vi "chooseKeeperPlay.vi"(8 "error in (no error)":errorcluster, 11 "Game in":refnum<class "Game.lvclass">) -> (0 "error out":errorcluster, 3 "Game out":refnum<class "Game.lvclass">)   [LabVIEW 2023, in "Game.lvclass"]
uses:
  Game.lvclass
  Game.lvclass/Game.ctl
  Team_class/Team.lvclass/Team.ctl
  HaltPlay_class/HaltPlay.lvclass
  ZigZagPlay_class/ZigZagPlay.lvclass
  TestPlay_class/TestPlay.lvclass
  TimeoutPlay_class/TimeoutPlay.lvclass
  Team_class/KeeperPlay.ctl
  Read KeeperTeam.vi
  Team_class/Read KeeperPlay.vi
  Read AllyRef.vi
  Team_class/Write KeeperPlay.vi
  Write AllyRef.vi
  Write KeeperTeam.vi
  Ally_class/Ally.lvclass
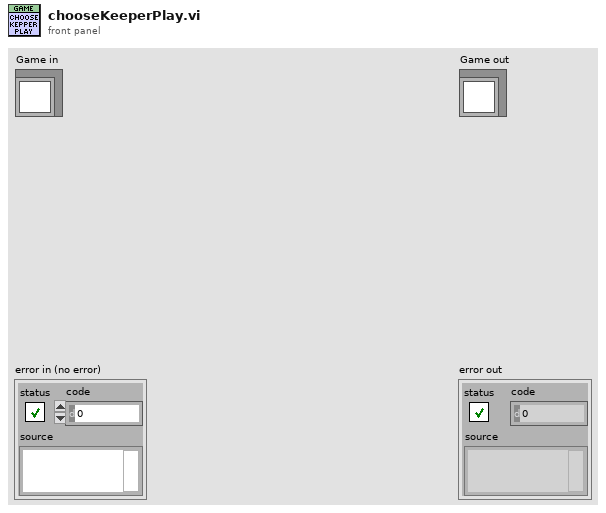
[diagram p1: front panel]
types:
  T1 = typedef "KeeperPlay.ctl" = enum16{"ZigZag", "Goto", "NormalGame", "KeeperPlay", "Halt", "Timeout", "PenaltyEnemy", "TestPlay"}
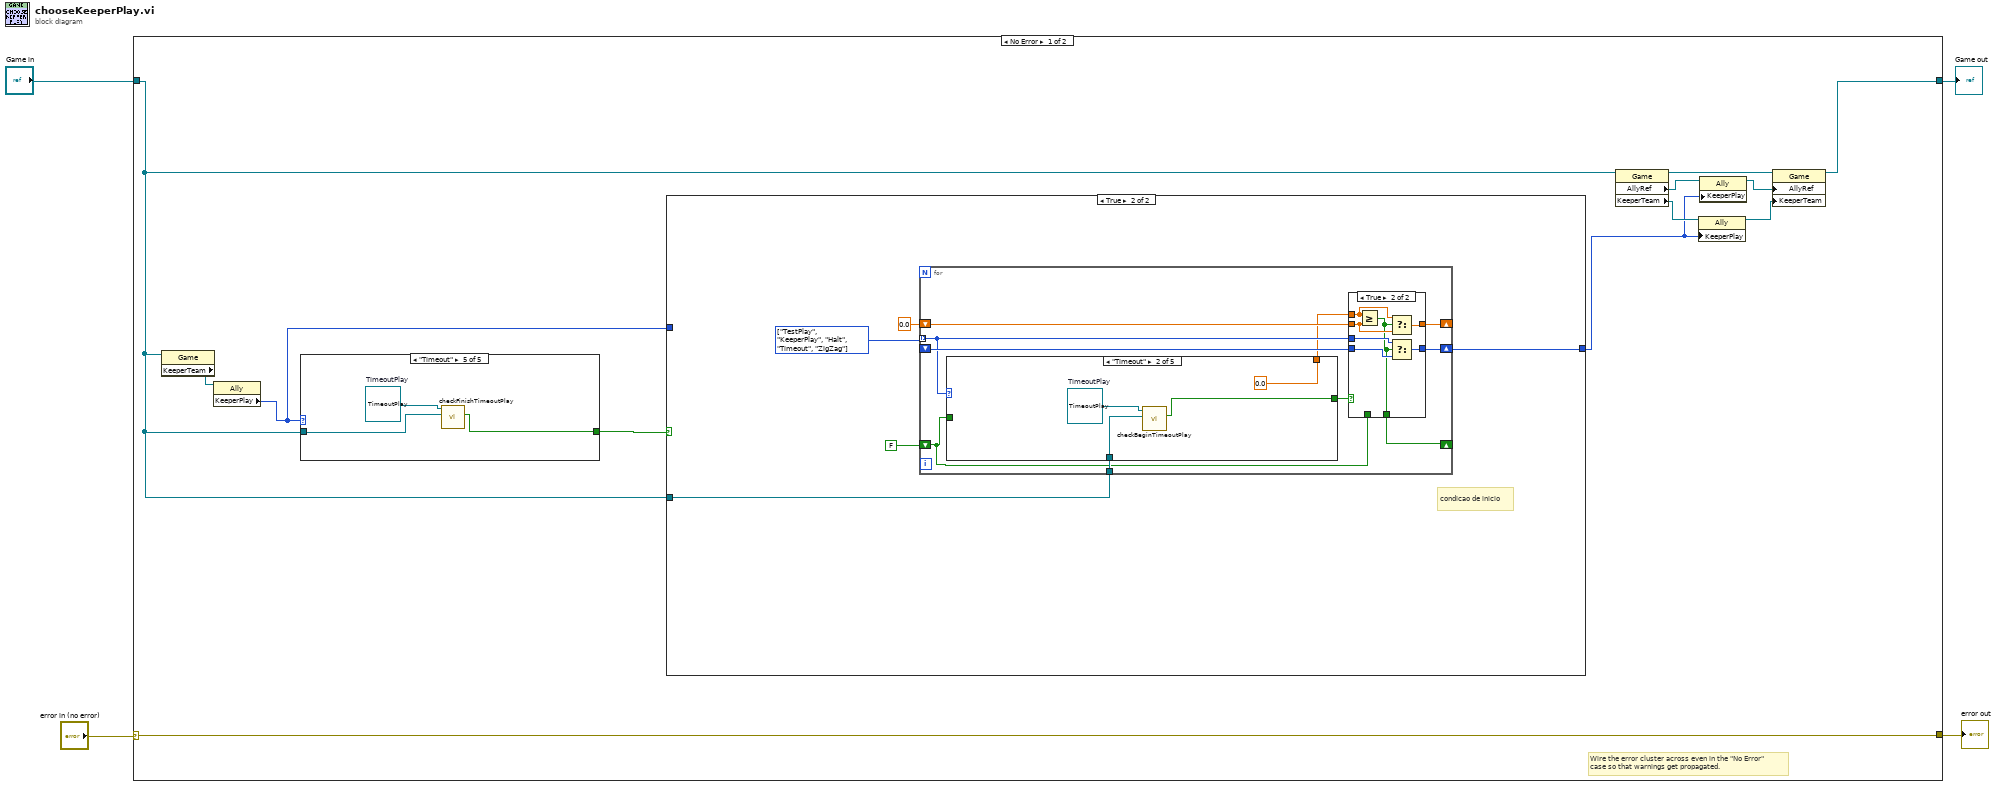
[diagram p0: block diagram]
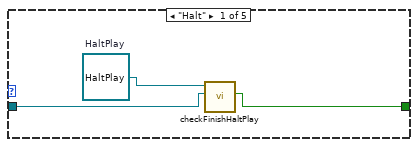
[diagram p2: hidden frame]
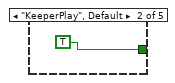
[diagram p3: hidden frame]
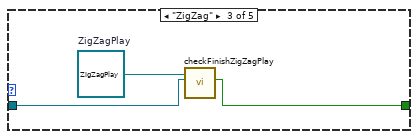
[diagram p4: hidden frame]
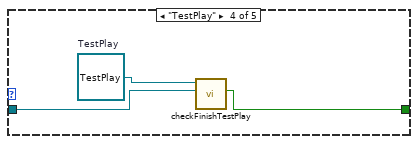
[diagram p5: hidden frame]
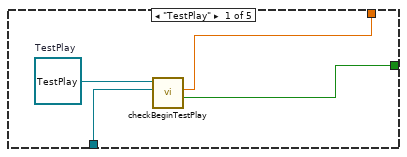
[diagram p7: hidden frame]
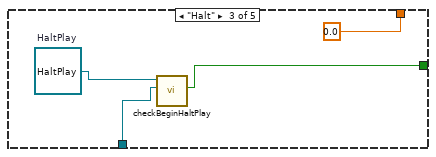
[diagram p8: hidden frame]
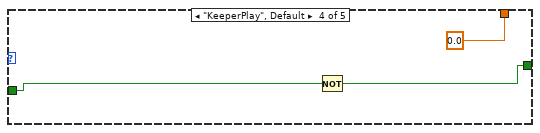
[diagram p9: hidden frame]
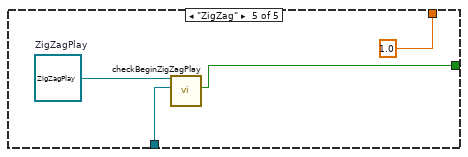
[diagram p10: hidden frame]
diagram:
  n1 = case shown="No Error" "error in (no error)" {
    selector: "error in (no error)" -> [w16 w76]
    tunnel: [w16 w76] -> w3
    tunnel: [w14 w75] -> w1
    tunnel: "Game in" -> [w8 w75]
    frame No Error {
      # "Wire the error cluster across even in the \"No Error\"\ncase so that warnings get propagated."
      n2 = property class="Game"(reference=w8) -> ("KeeperTeam"=w13:refnum<class "Ally.lvclass">)  [unwired: 1 in, 2 out]
      n3 = property class="Ally"(reference=w13) -> ("KeeperPlay"=w11:T1)  [unwired: 1 in, 2 out]
      n4 = case shown="\"Timeout\"" w11 {
        tunnel: [w17 TRUE w21 w24 w27] -> w12
        tunnel: w8 -> [w18 _ w22 w25 w28]
        frame "Halt" {
          w19 = refnum<class "HaltPlay.lvclass"> refnum  # HaltPlay
          n5 = call "checkFinishHaltPlay.vi"("Game"=w18, "HaltPlay in"=w19) -> ("Boolean"=w17:bool)  [unwired: 7 in, 2 out]
        }
        frame "KeeperPlay", Default {
        }
        frame "ZigZag" {
          w23 = refnum<class "ZigZagPlay.lvclass"> refnum  # ZigZagPlay
          n6 = call "checkFinishZigZagPlay.vi"("Game"=w22, "ZigZagPlay in"=w23) -> ("Boolean"=w21:bool)  [unwired: 7 in, 2 out]
        }
        frame "TestPlay" {
          w26 = refnum<class "TestPlay.lvclass"> refnum  # TestPlay
          n7 = call "checkFinishTestPlay.vi"("Game"=w25, "TestPlay in"=w26) -> ("Boolean"=w24:bool)  [unwired: 7 in, 2 out]
        }
        frame "Timeout" {
          w29 = refnum<class "TimeoutPlay.lvclass"> refnum  # TimeoutPlay
          n8 = call "checkFinishTimeoutPlay.vi"("Game"=w28, "TimeoutPlay in"=w29) -> ("Finish Timeout?"=w27:bool)  [unwired: 7 in, 2 out]
        }
      }
      n9 = case shown="True" w12 {
        tunnel: [w30 w34] -> w5
        tunnel: w11 -> [w30 _]
        tunnel: w8 -> [_ w33]
        frame False {
        }
        frame True {
          w31 = T1[] [enum."TestPlay", enum."KeeperPlay", enum."Halt", enum."Timeout", enum."ZigZag"] items=["ZigZag", "Goto", "NormalGame", "KeeperPlay", "Halt", "Timeout", "PenaltyEnemy", "TestPlay"] ("Array")
          # "condicao de inicio"
          n10 = for {
            tunnel: w31 -> [w41] mode=indexing
            shift-right: [w44] -> _
            shift-left: 0.0 -> [w43]
            shift-right: [w42] -> w34
            shift-left: _ -> [w45]
            tunnel: w33 -> [w38]
            shift-right: [w37] -> _
            shift-left: FALSE -> [w36]
            n11 = case shown="\"Timeout\"" w41 {
              tunnel: [w47 w51 w55 w60 w62] -> w40
              tunnel: [w46 0.0 0.0 0.0 1.0] -> w39
              tunnel: w38 -> [w48 w52 w56 _ w63]
              tunnel: w36 -> [_ _ _ w59 _]
              frame "TestPlay" {
                w49 = refnum<class "TestPlay.lvclass"> refnum  # TestPlay
                n12 = call "checkBeginTestPlay.vi"("Game"=w48, "TestPlay in"=w49) -> ("Test"=w47:bool, "Score out"=w46:dbl)  [unwired: 6 in, 2 out]
              }
              frame "Timeout" {
                w53 = refnum<class "TimeoutPlay.lvclass"> refnum  # TimeoutPlay
                n13 = call "checkBeginTimeoutPlay.vi"("Game"=w52, "TimeoutPlay in"=w53) -> ("BeginTimeout?"=w51:bool)  [unwired: 7 in, 2 out]
              }
              frame "Halt" {
                w57 = refnum<class "HaltPlay.lvclass"> refnum  # HaltPlay
                n14 = call "checkBeginHaltPlay.vi"("Game"=w56, "HaltPlay in"=w57) -> ("Boolean"=w55:bool)  [unwired: 7 in, 2 out]
              }
              frame "KeeperPlay", Default {
                n15 = Not(x=w59) -> (.not. x?=w60:bool)
              }
              frame "ZigZag" {
                w61 = refnum<class "ZigZagPlay.lvclass"> refnum  # ZigZagPlay
                n16 = call "checkBeginZigZagPlay.vi"("Game"=w63, "ZigZagPlay in"=w61) -> ("TestMode"=w62:bool)  [unwired: 7 in, 2 out]
              }
            }
            n17 = case shown="True" w40 {
              tunnel: w45 -> [w66 w71]
              tunnel: [w67 w74] -> w44
              tunnel: w43 -> [w67 w70]
              tunnel: w41 -> [_ w72]
              tunnel: [w66 w73] -> w42
              tunnel: w39 -> [_ w69]
              tunnel: [w65 w68] -> w37
              tunnel: w36 -> [w65 _]
              frame False {
              }
              frame True {
                n18 = Greater Or Equal?(x=w69, y=w70) -> (x >= y?=w68:bool)
                n19 = Select(t=w69, s=w68, f=w70) -> (s? t:f=w74:dbl)
                n20 = Select(t=w72, s=w68, f=w71) -> (s? t:f=w73:T1)
              }
            }
          }
        }
      }
      n21 = property class="Game"(reference=w8) -> (reference out=w15:refnum<class "Game.lvclass">, "AllyRef"=w7:refnum<class "Ally.lvclass">, "KeeperTeam"=w10:refnum<class "Ally.lvclass">)  [unwired: 1 in, 1 out]
      n22 = property class="Ally"(reference=w10, "KeeperPlay"=w5) -> (reference out=w9:refnum<class "Ally.lvclass">)  [unwired: 1 in, 1 out]
      n23 = property class="Ally"(reference=w7, "KeeperPlay"=w5) -> (reference out=w6:refnum<class "Ally.lvclass">)  [unwired: 1 in, 1 out]
      n24 = property class="Game"(reference=w15, "AllyRef"=w6, "KeeperTeam"=w9) -> (reference out=w14:refnum<class "Game.lvclass">)  [unwired: 1 in, 1 out]
    }
    frame Error {
    }
  }
  "error out" <- w3
  "Game out" <- w1
